vi "_scriptEditor Parse CSM State.vi"(11 "single-line text":string="status@asdfasf >> abcdef@xaef -><register>") -> (0 "Msg Type":T2=enum."Message", 2 "comments":T1, 3 "Array":string[](array[string])=["status@asdfasf ", ">>", " abcdef@xaef ", "->", "<register>"])   [LabVIEW 2017]
uses:
  def-message type.ctl
  <vilib>/regexp/Match Regular Expression.xnode
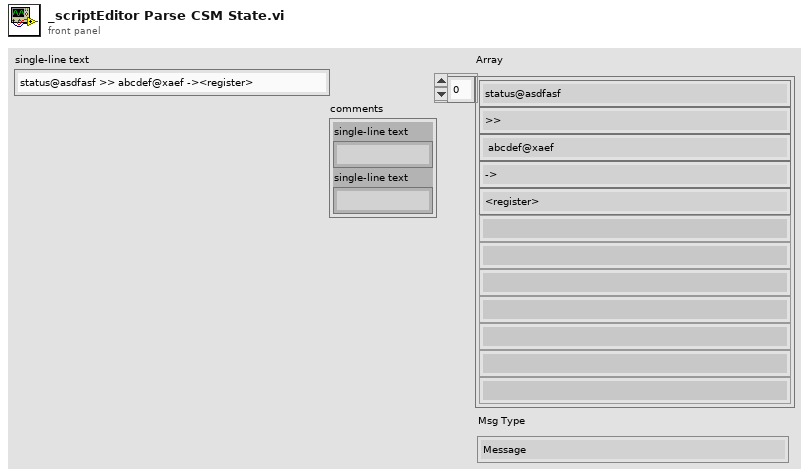
[diagram p1: front panel]
types:
  T1 = cluster{"single-line text":string, "single-line text":string}
  T2 = typedef "def-message type.ctl" = enum16{"State", "Message", "Broadcast", "Registration"}
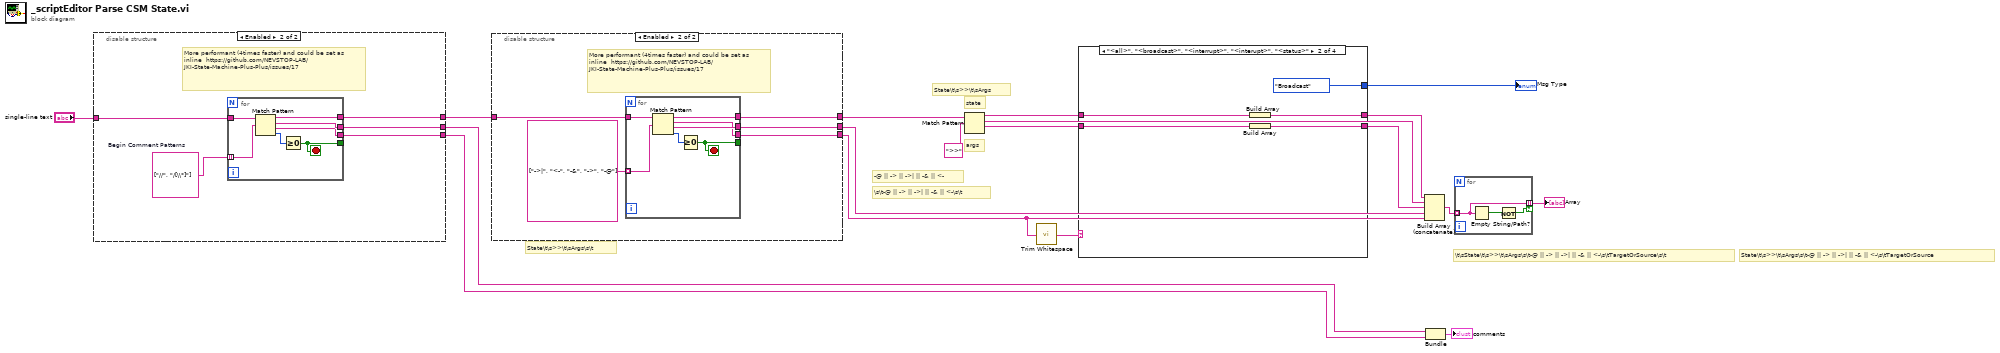
[diagram p0: block diagram]
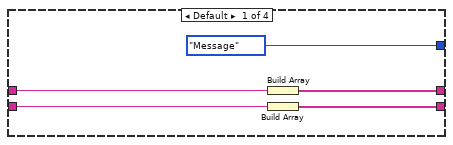
[diagram p2: hidden frame]
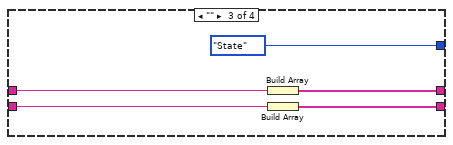
[diagram p3: hidden frame]
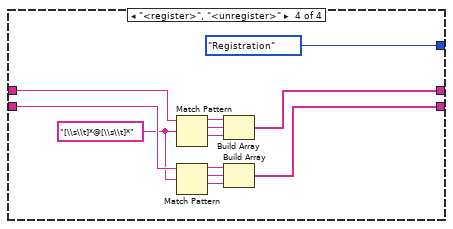
[diagram p4: hidden frame]
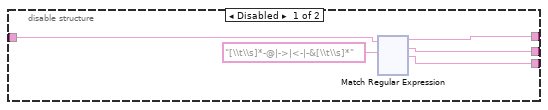
[diagram p5: hidden frame]
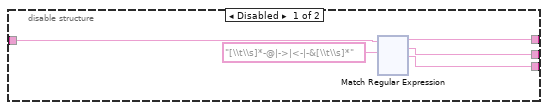
[diagram p6: hidden frame]
diagram:
  # "\\t\\sState\\t\\s>>\\t\\sArgs\\s\\t-@ || -> || ->| || -& || <-\\s\\tTargetOrSource\\s\\t"
  # "-@ || -> || ->| || -& || <-"
  # "\\s\\t-@ || -> || ->| || -& || <-\\s\\t"
  # "State\\t\\s>>\\t\\sArgs"
  # "State\\t\\s>>\\t\\sArgs\\s\\t"
  # "State\\t\\s>>\\t\\sArgs\\s\\t-@ || -> || ->| || -& || <-\\s\\tTargetOrSource"
  # "args"
  # "state"
  n1 = disable-structure shown="Enabled" {
    disable-tunnel: [w22 w141] -> w18
    disable-tunnel: [w21 w140] -> w3
    disable-tunnel: [w20 w139] -> w2
    disable-tunnel: "single-line text" -> [w19 w142]
    frame Disabled {
      n2 = xnode "Match Regular Expression"("input string"=w19, "regular expression"="[\\t\\s]*-@|->|<-|-&[\\t\\s]*") -> ("before match"=w22:string, "whole match"=w21:string, "after match"=w20:string)  [unwired: 4 in, 2 out]
    }
    frame Enabled {
      w138 = string[] ["//", "/[\\*]"]  # Begin Comment Patterns
      # "More performant (4times faster) and could be set as inline  https://github.com/NEVSTOP-LAB/JKI-State-Machine-Plus-Plus/issues/17"
      n3 = for {
        tunnel: w142 -> [w149]
        tunnel: w138 -> [w148] mode=indexing
        tunnel: [w146] -> _
        tunnel: [w145] -> w141
        tunnel: [w144] -> w140
        tunnel: [w143] -> w139
        stop <- w146 stop-if-true
        n4 = Match Pattern(string=w149, regular expression=w148) -> (before substring=w145:string, match substring=w144:string, after substring=w143:string, offset past match=w147:i32)  [unwired: 1 in]
        n5 = Greater Or Equal To 0?(x=w147) -> (x >= 0?=w146:bool)
      }
    }
  }
  n6 = disable-structure shown="Enabled" {
    disable-tunnel: [w153 w271] -> w13
    disable-tunnel: [w152 w270] -> w14
    disable-tunnel: [w151 w269] -> w6
    disable-tunnel: w18 -> [w150 w273]
    frame Disabled {
      n7 = xnode "Match Regular Expression"("input string"=w150, "regular expression"="[\\t\\s]*-@|->|<-|-&[\\t\\s]*") -> ("before match"=w153:string, "whole match"=w152:string, "after match"=w151:string)  [unwired: 4 in, 2 out]
    }
    frame Enabled {
      # "More performant (4times faster) and could be set as inline  https://github.com/NEVSTOP-LAB/JKI-State-Machine-Plus-Plus/issues/17"
      n8 = for {
        tunnel: w273 -> [w280]
        tunnel: string[] ["->|", "<-", "-&", "->", "-@"] -> [w279] mode=indexing
        tunnel: [w277] -> _
        tunnel: [w276] -> w271
        tunnel: [w275] -> w270
        tunnel: [w274] -> w269
        stop <- w277 stop-if-true
        n9 = Match Pattern(string=w280, regular expression=w279) -> (before substring=w276:string, match substring=w275:string, after substring=w274:string, offset past match=w278:i32)  [unwired: 1 in]
        n10 = Greater Or Equal To 0?(x=w278) -> (x >= 0?=w277:bool)
      }
    }
  }
  n11 = Match Pattern(string=w13, regular expression=">>") -> (before substring=w8:string, match substring=w11:string, after substring=w10:string)  [unwired: 1 in, 1 out]
  n12 = call <vilib>:"Trim Whitespace.vi"("string"=w6) -> ("trimmed string"=w5:string)  [unwired: 1 in]
  n13 = case shown="\"<all>\", \"<broadcast>\", \"<interrupt>\", \"<interupt>\", \"<status>\"" w5 {
    tunnel: w10 -> [w284 w289 w294 w299]
    tunnel: [w283 w288 w293 w298] -> w9
    tunnel: w8 -> [w285 w290 w295 w307]
    tunnel: [w282 w287 w292 w303] -> w7
    tunnel: [def-message_type."Message" ("Msg Type") def-message_type."Broadcast" ("Msg Type") def-message_type."State" ("Msg Type") def-message_type."Registration" ("Msg Type")] -> w4
    frame Default {
      n14 = Build Array(w285) -> (w282:string[])
      n15 = Build Array(w284) -> (w283:string[])
    }
    frame "<all>", "<broadcast>", "<interrupt>", "<interupt>", "<status>" {
      n16 = Build Array(w290) -> (w287:string[])
      n17 = Build Array(w289) -> (w288:string[])
    }
    frame "" {
      n18 = Build Array(w295) -> (w292:string[])
      n19 = Build Array(w294) -> (w293:string[])
    }
    frame "<register>", "<unregister>" {
      w296 = "[\\s\\t]*@[\\s\\t]*" ("regular expression")
      n20 = Match Pattern(string=w307, regular expression=w296) -> (before substring=w306:string, match substring=w305:string, after substring=w304:string)  [unwired: 1 in, 1 out]
      n21 = Match Pattern(string=w299, regular expression=w296) -> (before substring=w300:string, match substring=w301:string, after substring=w302:string)  [unwired: 1 in, 1 out]
      n22 = Build Array(w306, w305, w304) -> (w303:string[])
      n23 = Build Array(w300, w301, w302) -> (w298:string[])
    }
  }
  "Msg Type" <- w4
  n24 = Build Array (concatenate)(w7, w11, w9, w14, w6) -> (w16:string[])
  n25 = Bundle("single-line text"=w3, "single-line text"=w2) -> (→"comments":T1)  [unwired: 1 in]
  n26 = for {
    tunnel: [w310] -> w15 mode=indexing if=w308
    tunnel: w16 -> [w310] mode=indexing
    n27 = Empty String/Path?(string/path=w310) -> (empty?=w309:bool)
    n28 = Not(x=w309) -> (.not. x?=w308:bool)
  }
  "Array" <- w15
